vi "Sequence Experiment.getAll.vi"(8 "error in (no error)":errorcluster, 11 "Sequence Experiment":refnum<class "Sequence Experiment.lvclass">) -> (0 "error out":errorcluster, 2 "getAll":T1, 3 "Sequence Experiment out":refnum<class "Sequence Experiment.lvclass">)   [LabVIEW 2019, in "Sequence Experiment.lvclass"]
uses:
  Sequence Experiment.lvclass
  Typedefs/Sequence Experiment.getAll--Cluster.ctl
  7fbd5c49-7ee6-445a-8372-f8319484267f.vi
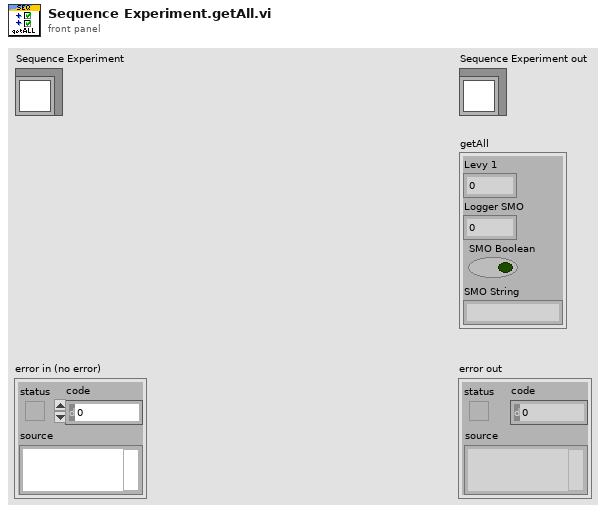
[diagram p1: front panel]
types:
  T1 = typedef "Sequence Experiment.lvclass/Sequence Experiment.getAll--Cluster.ctl" = cluster{"Levy 1":dbl, "Logger SMO":dbl, "SMO Boolean":bool, "SMO String":string}
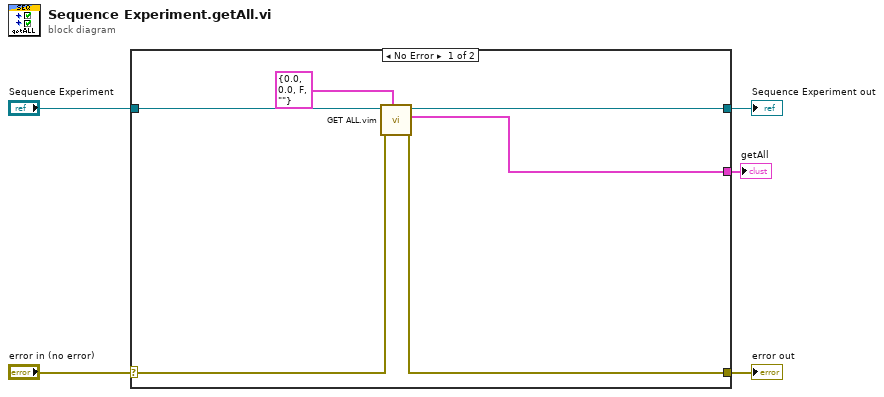
[diagram p0: block diagram]
diagram:
  n1 = case shown="No Error" "error in (no error)" {
    selector: "error in (no error)" -> [w9 w13]
    tunnel: [w7 w13] -> w4
    tunnel: [w10 w12] -> w2
    tunnel: "Sequence Experiment" -> [w11 w12]
    tunnel: [w6 _] -> w1
    frame No Error {
      n2 = call "GET ALL.vim"("type"=T1 {"Levy 1"=0.0, "Logger SMO"=0.0, "SMO Boolean"=FALSE, "SMO String"=""} ("getAll"), "error in (no error)"=w9, "Instrument in"=w11) -> ("error out"=w7:errorcluster, "getAll"=w6:T1, "Instrument out"=w10:refnum<class "Sequence Experiment.lvclass">)  [unwired: 6 in]
    }
    frame Error {
    }
  }
  "error out" <- w4
  "Sequence Experiment out" <- w2
  "getAll" <- w1
